vi "430_RS232_Command.vi"(3 "error in (no error)":errorcluster, 5 "Command":string, 6 "VISA resource name":refnum<visa-resource-name>="COM1") -> (0 "error out":errorcluster, 1 "bytes written":i32, 2 "VISA resource name out":refnum<visa-resource-name>="COM1")   [LabVIEW 2017]
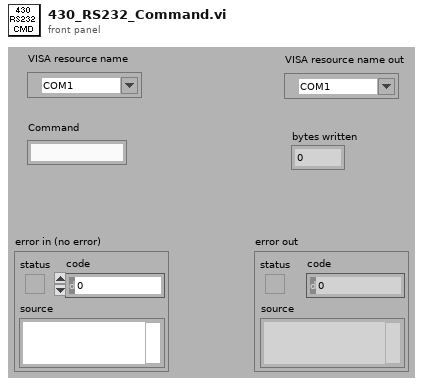
[diagram p1: front panel]
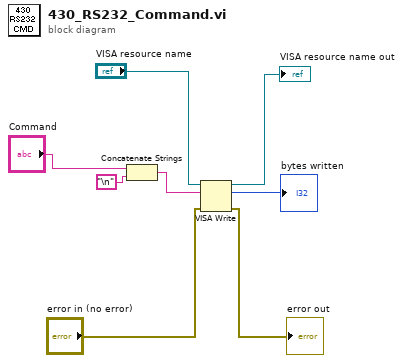
[diagram p0: block diagram]
diagram:
  n1 = Concatenate Strings("Command", "\n") -> (w4:string)
  n2 = VISA Write(VISA resource name="VISA resource name", write buffer=w4, error in (no error)="error in (no error)") -> (VISA resource name out=→"VISA resource name out":refnum<visa-resource-name>, return count=→"bytes written":u32, error out=→"error out":errorcluster)
